vi "Get_Horizontal_Scale.vi"(7 "error in (no error)":errorcluster, 10 "VISA resource name":refnum<visa-resource-name>="Master_Oscilloscope") -> (0 "error out":errorcluster, 2 "Horizontal_Parameters":string[](array[string]), 3 "VISA resource name out":refnum<visa-resource-name>)   [LabVIEW 2020]
panel:
  out "Sampling Frequency":string
  out "Epoch Value":string
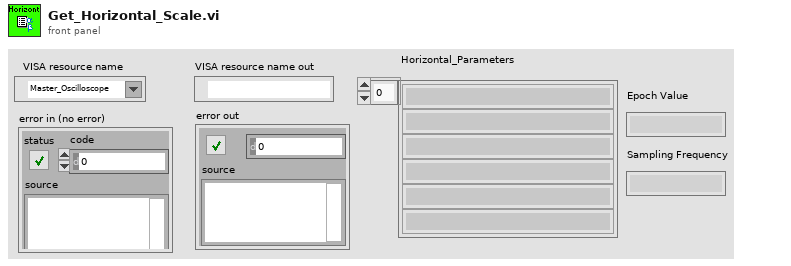
[diagram p1: front panel]
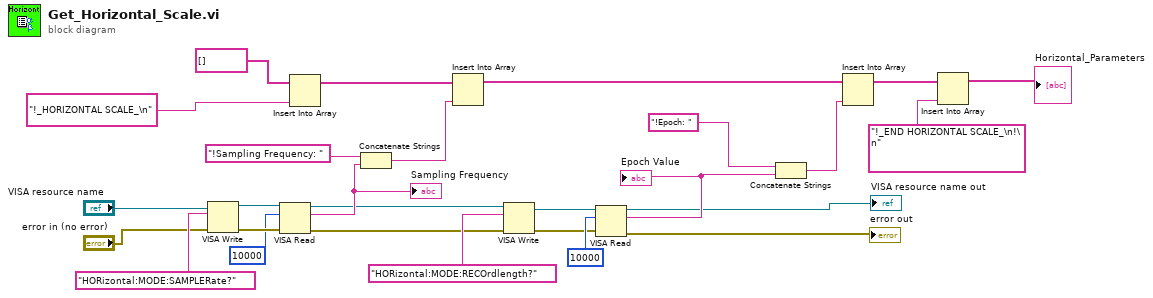
[diagram p0: block diagram]
diagram:
  n1 = VISA Write(VISA resource name="VISA resource name", write buffer="HORizontal:MODE:SAMPLERate?", error in (no error)="error in (no error)") -> (VISA resource name out=w19:refnum<visa-resource-name>, error out=w20:errorcluster)  [unwired: 1 out]
  n2 = VISA Read(VISA resource name=w19, byte count=u32 10000, error in (no error)=w20) -> (VISA resource name out=w15:refnum<visa-resource-name>, read buffer=w16:string, error out=w14:errorcluster)  [unwired: 1 out]
  "Sampling Frequency" <- w16
  n3 = Insert Into Array(array=string[] [], new element="!_HORIZONTAL SCALE_\n") -> (w7:string[])  [unwired: 1 in]
  n4 = Concatenate Strings("!Sampling Frequency: " ("string"), w16) -> (w6:string)
  n5 = Insert Into Array(array=w7, new element=w6) -> (w5:string[])  [unwired: 1 in]
  n6 = VISA Write(VISA resource name=w15, write buffer="HORizontal:MODE:RECOrdlength?", error in (no error)=w14) -> (VISA resource name out=w25:refnum<visa-resource-name>, error out=w24:errorcluster)  [unwired: 1 out]
  n7 = VISA Read(VISA resource name=w25, byte count=u32 10000, error in (no error)=w24) -> (VISA resource name out=→"VISA resource name out":refnum<visa-resource-name>, read buffer=w22:string, error out=→"error out":errorcluster)  [unwired: 1 out]
  "Epoch Value" <- w22
  n8 = Concatenate Strings("!Epoch: " ("string"), w22) -> (w4:string)
  n9 = Insert Into Array(array=w5, new element=w4) -> (w3:string[])  [unwired: 1 in]
  n10 = Insert Into Array(array=w3, new element="!_END HORIZONTAL SCALE_\n!\n" ("new element/subarray")) -> (→"Horizontal_Parameters":string[])  [unwired: 1 in]
